vi "Global 1.vi"() -> ()   [LabVIEW 2017]
panel:
  out "Position#":dbl
  out "DistanceSwitch":dbl
  out "DistanceScaleBas":dbl
  out "DistanceScaleHaut":dbl
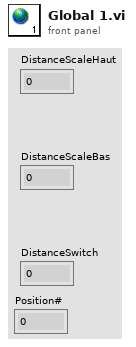
[diagram p1: front panel]
diagram:
